vi "set up imaqdx aquisition.vi"(8 "error in (no error)":errorcluster, 11 "camera name":T2) -> (0 "error out":errorcluster, 1 "camera image is 8 bit":bool, 2 "camera image":T3, 3 "imaqdx session":T2 caption="Session Out")   [LabVIEW 2013]
uses:
  <vilib>/vision/Image Controls.llb/IMAQ Image.ctl
  <vilib>/userdefined/High Color/IMAQdx.ctl
  <vilib>/vision/driver/NI_Vision_Acquisition_Software.lvlib
  <resource>/objmgr/imaqdx.rc
panel:
  out "Image Type":T1 items=["Grayscale (U8)", "Grayscale (I16)", "Grayscale (SGL)", "Complex (CSG)", "RGB (U32)", "HSL (U32)", "RGB (U64)", "Grayscale (U16)"]
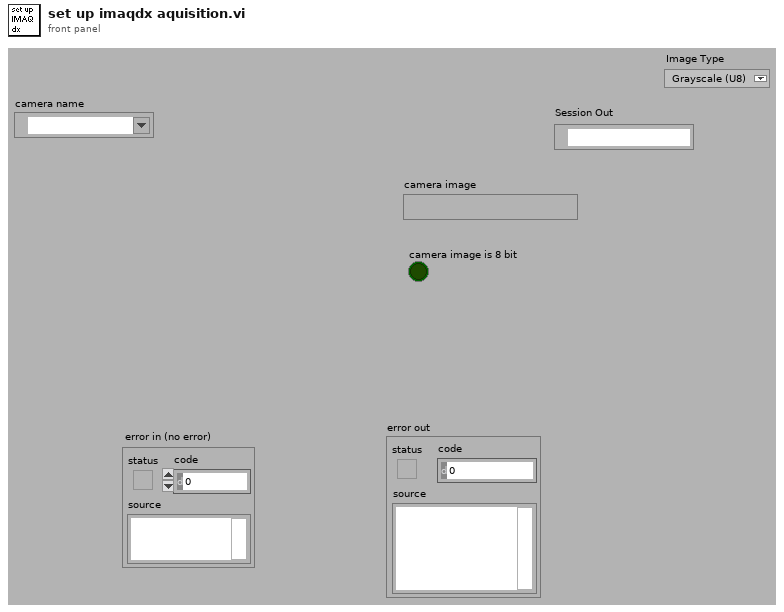
[diagram p1: front panel]
types:
  T1 = typedef "Image Type" = u32
  T2 = typedef "IMAQdx.ctl" = refnum<k21>
  T3 = typedef "IMAQ Image.ctl" = refnum<image>
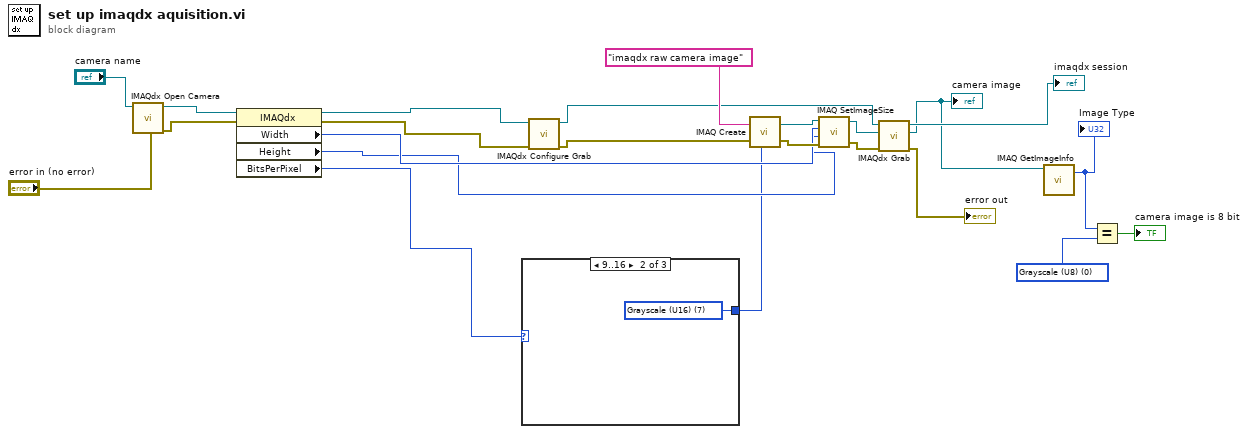
[diagram p0: block diagram]
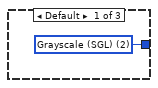
[diagram p2: hidden frame]
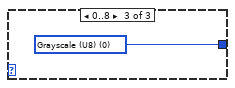
[diagram p3: hidden frame]
diagram:
  w15 = u32 0 items=["Grayscale (U8)", "Grayscale (I16)", "Grayscale (SGL)", "Complex (CSG)", "RGB (U32)", "HSL (U32)", "RGB (U64)"] ("Image Parameters : Image Type")
  n1 = call <vilib>:"IMAQdx Open Camera.vi"("error in"="error in (no error)", "Session In"="camera name") -> ("error out"=w11:errorcluster, "Session Out"=w10:T2)  [unwired: 8 in]
  n2 = property class="IMAQdx"(reference=w10, error in=w11) -> (reference out=w22:T2, error out=w23:errorcluster, "Width"=w17:u32, "Height"=w16:u32, "BitsPerPixel"=w2:u32)
  n3 = case shown="9..16" w2 {
    tunnel: [w24 w25 w26] -> w1
    frame Default {
      w24 = T1 2 items=["Grayscale (U8)", "Grayscale (I16)", "Grayscale (SGL)", "Complex (CSG)", "RGB (U32)", "HSL (U32)", "RGB (U64)", "Grayscale (U16)"] ("Image Type")
    }
    frame 9..16 {
      w25 = T1 7 items=["Grayscale (U8)", "Grayscale (I16)", "Grayscale (SGL)", "Complex (CSG)", "RGB (U32)", "HSL (U32)", "RGB (U64)", "Grayscale (U16)"] ("Image Type")
    }
    frame 0..8 {
      w26 = T1 0 items=["Grayscale (U8)", "Grayscale (I16)", "Grayscale (SGL)", "Complex (CSG)", "RGB (U32)", "HSL (U32)", "RGB (U64)", "Grayscale (U16)"] ("Image Type")
    }
  }
  n4 = call <vilib>:"IMAQdx Configure Grab.vi"("error in"=w23, "Session In"=w22) -> ("error out"=w21:errorcluster, "Session Out"=w7:T2)  [unwired: 8 in]
  n5 = call "IMAQ Create"("Image Name"="imaqdx raw camera image", "Image Type"=w1, "error in (no error)"=w21) -> ("New Image"=w18:T3, "error out"=w19:errorcluster)  [unwired: 2 in]
  n6 = call "IMAQ SetImageSize"("error in (no error)"=w19, "Y Resolution"=w16, "X Resolution"=w17, "Image"=w18) -> ("error out"=w9:errorcluster, "Image Out"=w8:T3)  [unwired: 1 in]
  n7 = call <vilib>:"IMAQdx Grab.vi"("error in"=w9, "Image In"=w8, "Session In"=w7) -> ("error out"=→"error out":errorcluster, "Image Out"=w4:T3, "Session Out"=→"imaqdx session":T2)  [unwired: 5 in, 1 out]
  "camera image" <- w4
  n8 = call "IMAQ GetImageInfo"("Image"=w4) -> ("Image Type"=w3:T1)  [unwired: 3 in, 7 out]
  "Image Type" <- w3
  n9 = Equal?(x=w3, y=w15) -> (x = y?=→"camera image is 8 bit":bool)
